vi "Write val.vi"(8 "error in (no error)":errorcluster, 10 "val":dbl, 11 "Switch DBL in":refnum<class "Switch DBL.lvclass">) -> (0 "error out":errorcluster, 3 "Switch DBL out":refnum<class "Switch DBL.lvclass">)   [LabVIEW 2015, in "Sequence Composition.lvlib" / "Switch DBL.lvclass"]
uses:
  Switch DBL.lvclass
  Switch DBL.lvclass/Switch DBL.ctl
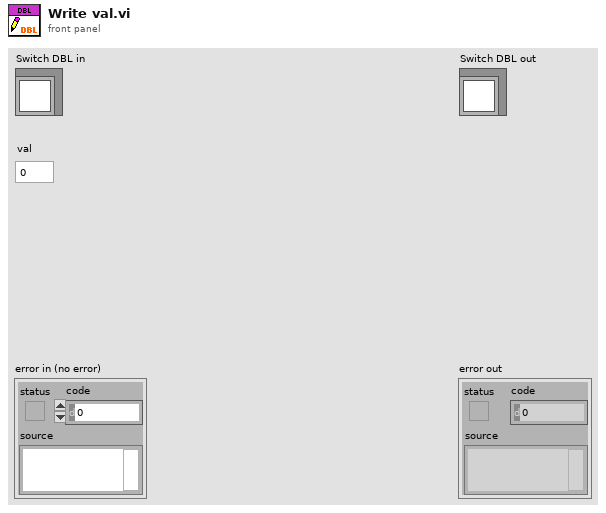
[diagram p1: front panel]
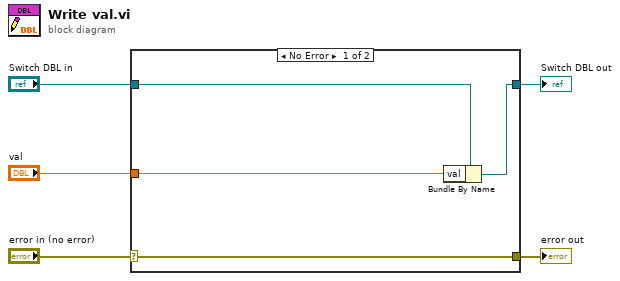
[diagram p0: block diagram]
diagram:
  n1 = case shown="No Error" "error in (no error)" {
    selector: "error in (no error)" -> [w9 w10]
    tunnel: [w9 w10] -> w4
    tunnel: [w7 w11] -> w2
    tunnel: "Switch DBL in" -> [w8 w11]
    tunnel: "val" -> [w6 _]
    frame No Error {
      n2 = Bundle By Name(cluster=w8, "val"=w6) -> (w7:refnum<class "Switch DBL.lvclass">)
    }
    frame Error {
    }
  }
  "error out" <- w4
  "Switch DBL out" <- w2
